vi "CST.vi"(0 "System no.":i32=1 min=1 max=4 step=1, 2 "Axis ID's":string[](array[string]), 3 "Stage names":string[](array[string]), 5 "error in":errorcluster) -> (19 "error out":errorcluster)   [LabVIEW 2020]
doc: "Assigns axes to stages and queries ERR?. With this command the stage assignment of the connected axes can be changed. Valid stage names can be listed with VST?.vi.\nAxes assignment is written to volatile memory only and will be lost after restarting the controller. To assign the axes permanently, please use the WPA command.\n\nC-877, C-884, E-872, E-873: Command is available via USB interface only.\n\nC-891: : Command is available via USB interface only. Axes assignment will be written to non volatile memory and will be available even after restarting the controller. Controller may reboot while CST command is in progress.\n\nE-761: The settings are automatically written to non-volatile memory. Valid stage names are \"ID-STAGE\" for configured axes (a stage should be connected) and \"NOSTAGE\" for non-configured axes (no stage should be connected). The axis configuration as \"ID-STAGE\" is required before you can address any move command to this axis (i.e. to the connected stage).\n\nC-867, E-871, Mercury_GCS: Command is available via USB, USB DaisyChain or RS232 DaisyChain interface only.\n\nC-887, F-206, M-8X0: Only for GCS syntax version = GCS 2.0 or higher (check with CSV?.vi. If CSV?.vi is not supported, syntax version is GCS 1.0). Only valid for separate axes A and/or B.\n\nPollux: See HydraPollux_GCS_DLL Manual for specialities of the Pollux controller family regarding stage name settings."
panel:
  # "Assigns axes to stages and queries for ERR?. With this command the stage \nassignment of the connected axes can be changed. Valid stage names can be \nlisted with VST?.vi."
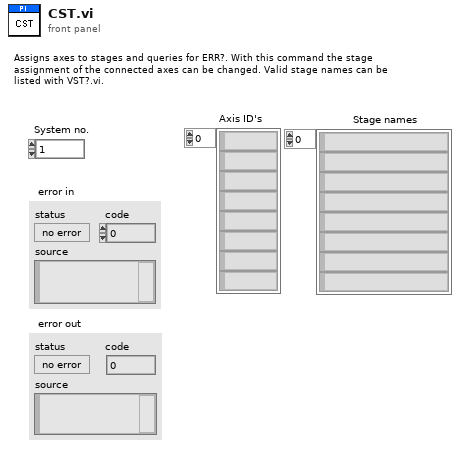
[diagram p1: front panel]
types:
  T1 = enum16{"Disable error check", "Force error check", "Use global settings"}
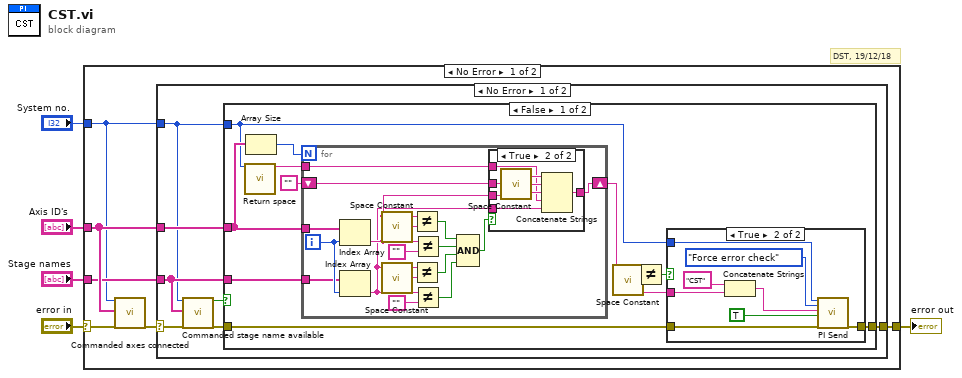
[diagram p0: block diagram]
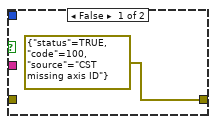
[diagram p2: hidden frame]
diagram:
  # "DST, 19/12/18"
  n1 = case shown="No Error" "error in" {
    selector: "error in" -> [w6 w65]
    tunnel: "Axis ID's" -> [w11 _]
    tunnel: [w10 w65] -> w4
    tunnel: "Stage names" -> [w9 _]
    tunnel: "System no." -> [w8 _]
    frame No Error {
      n2 = call "Commanded axes connected.vi"("System no."=w8, "Commanded axes"=w11, "error in"=w6) -> ("error out"=w7:errorcluster)  [unwired: 16 out]
      n3 = case shown="No Error" w7 {
        selector: w7 -> [w13 w64]
        tunnel: w11 -> [w18 _]
        tunnel: [w17 w64] -> w10
        tunnel: w9 -> [w16 _]
        tunnel: w8 -> [w12 _]
        frame No Error {
          n4 = call "Commanded stage name available.vi"("System no."=w12, "Commanded stages"=w16, "error in"=w13) -> ("Controller error"=w14:bool, "error out"=w15:errorcluster)  [unwired: 15 out]
          n5 = case shown="False" w14 {
            tunnel: w18 -> [w29 _]
            tunnel: w12 -> [w21 _]
            tunnel: [w19 w63] -> w17
            tunnel: w16 -> [w23 _]
            tunnel: w15 -> [w22 w63]
            frame False {
              n6 = call "Return space.vi"("System no."=w21) -> ("String out"=w20:string)  [unwired: 1 in, 17 out]
              n7 = Array Size(array=w29) -> (size(s)=w24:i32)
              n8 = for {
                N: w24 -> [_]
                tunnel: w29 -> [w44]
                shift-right: [w53] -> w26
                shift-left: "" -> [w54]
                tunnel: w23 -> [w42]
                tunnel: w20 -> [w40]
                i -> [w43]
                n9 = Index Array(array=w44, index=w43) -> (element=w52:string)
                n10 = Index Array(array=w42, index=w43) -> (element=w41:string)
                n11 = call <vilib>:"Space Constant.vi"() -> ("String"=w55:string)
                n12 = call <vilib>:"Space Constant.vi"() -> ("String"=w50:string)
                n13 = Not Equal?(x=w52, y=w55) -> (x != y?=w48:bool)
                n14 = Not Equal?(x=w41, y=w50) -> (x != y?=w46:bool)
                n15 = Not Equal?(x=w52, y="") -> (x != y?=w47:bool)
                n16 = Not Equal?(x=w41, y="") -> (x != y?=w45:bool)
                n17 = Compound Arithmetic op=AND(w48, w47, w46, w45) -> (w39:bool)
                n18 = case shown="True" w39 {
                  tunnel: w54 -> [w56 w62]
                  tunnel: w52 -> [_ w59]
                  tunnel: [w56 w61] -> w53
                  tunnel: w41 -> [_ w58]
                  tunnel: w40 -> [_ w57]
                  frame False {
                  }
                  frame True {
                    n19 = call <vilib>:"Space Constant.vi"() -> ("String"=w60:string)
                    n20 = Concatenate Strings(w62, w60, w59, w57, w58) -> (w61:string)
                  }
                }
              }
              n21 = call <vilib>:"Space Constant.vi"() -> ("String"=w27:string)
              n22 = Not Equal?(x=w26, y=w27) -> (x != y?=w25:bool)
              n23 = case shown="True" w25 {
                tunnel: w26 -> [_ w36]
                tunnel: w22 -> [_ w34]
                tunnel: w21 -> [_ w33]
                tunnel: [errorcluster {"status"=TRUE, "code"=100, "source"="CST missing axis ID"} ("error out") w32] -> w19
                frame False {
                }
                frame True {
                  n24 = Concatenate Strings("CST", w36) -> (w35:string)
                  n25 = call "PI Send.vi"("System no."=w33, "Error check settings"=T1."Force error check", "String to send"=w35, "Attach termination char.?"=TRUE ("Attach Linefeed?"), "error in"=w34) -> ("error out"=w32:errorcluster)  [unwired: 1 in, 13 out]
                }
              }
            }
            frame True {
            }
          }
        }
        frame Error {
        }
      }
    }
    frame Error {
    }
  }
  "error out" <- w4
